vi "Change ListBox FocusRow.vi"(8 "error in (no error)":errorcluster, 10 "Variation":i32, 11 "LstBox Refnum":refnum<vi>) -> (0 "error out":errorcluster, 3 "Listbox Reference out":refnum<vi>)   [LabVIEW 2015]
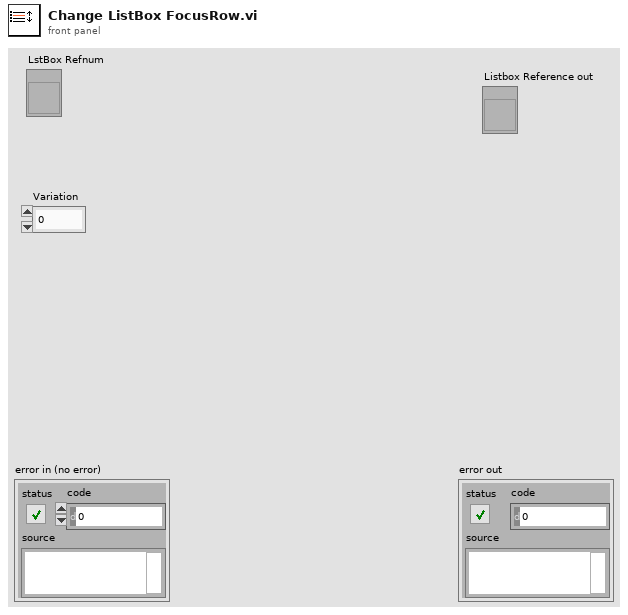
[diagram p1: front panel]
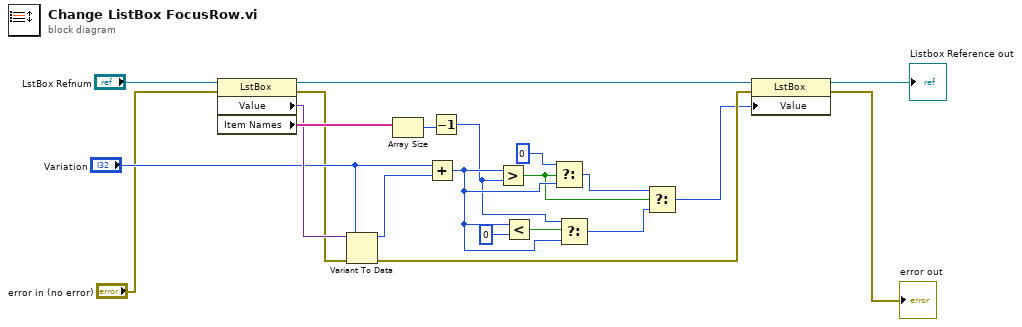
[diagram p0: block diagram]
diagram:
  n1 = property class="LstBox"(reference="LstBox Refnum", error in="error in (no error)") -> (reference out=w20:refnum<vi>, error out=w15:errorcluster, "Value"=w18:variant, "Item Names"=w21:string[])
  n2 = Variant To Data(error in=w15, type="Variation", Variant=w18) -> (data=w16:i32, error out=w14:errorcluster)
  n3 = Array Size(array=w21) -> (size(s)=w2:i32)
  n4 = Add(x="Variation", y=w16) -> (x+y=w9:i32)
  n5 = Decrement(x=w2) -> (x-1=w1:i32)
  n6 = Greater?(x=w9, y=w1) -> (0:w8:bool)
  n7 = Less?(x=w9, y=0) -> (x < y?=w10:bool)
  n8 = Select(t=0, s=w8, f=w9) -> (s? t:f=w7:i32)
  n9 = Select(t=w1, s=w10, f=w9) -> (s? t:f=w6:i32)
  n10 = Select(t=w7, s=w8, f=w6) -> (s? t:f=w5:i32)
  n11 = property class="LstBox"(reference=w20, error in=w14, "Value"=w5) -> (reference out=→"Listbox Reference out":refnum<vi>, error out=→"error out":errorcluster)
